vi "Get_Profile_paths.vi"(8 "error in (no error)":errorcluster, 10 "Target?":bool, 11 "OSArch":string) -> (0 "error out":errorcluster, 3 "profileDestPath":string)   [LabVIEW 2020, in "SEECD System Explorer.lvlib"]
uses:
  SEECD System Explorer.lvlib
  Applications/Utilities/ECAT Files.ctl
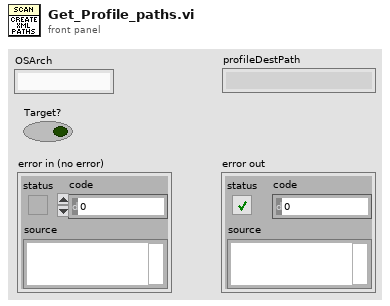
[diagram p1: front panel]
types:
  T1 = typedef "SEECD System Explorer.lvlib/ECAT Files.ctl" = enum16{"niECATLVProvider.mxx", "indcomecat.chm", "Providers DD", "Shared DD"}
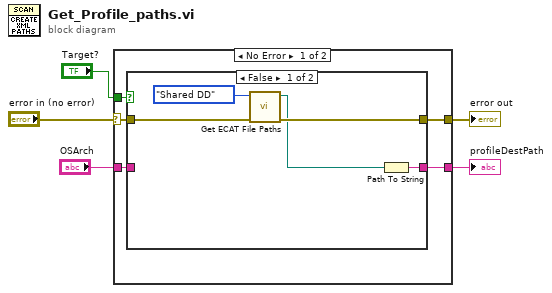
[diagram p0: block diagram]
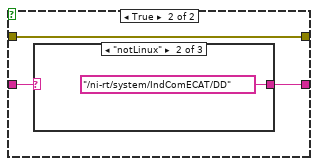
[diagram p2: hidden frame]
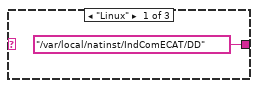
[diagram p3: hidden frame]
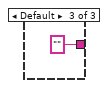
[diagram p4: hidden frame]
diagram:
  n1 = case shown="No Error" "error in (no error)" {
    selector: "error in (no error)" -> [w7 w22]
    tunnel: "OSArch" -> [w10 _]
    tunnel: [w6 w22] -> w4
    tunnel: "Target?" -> [w9 _]
    tunnel: [w8 _] -> w1
    frame No Error {
      n2 = case shown="False" w9 {
        tunnel: w10 -> [_ w18]
        tunnel: [w15 w17] -> w8
        tunnel: w7 -> [w14 w16]
        tunnel: [w13 w16] -> w6
        frame False {
          n3 = call "Get ECAT File Paths.vi"("error in"=w14, "ECAT File"=ECAT_Files."Shared DD") -> ("error out"=w13:errorcluster, "File Path"=w11:path)  [unwired: 8 in]
          n4 = Path To String(path=w11) -> (string=w15:string)
        }
        frame True {
          n5 = case shown="\"notLinux\"" w18 {
            tunnel: ["/var/local/natinst/IndComECAT/DD" "/ni-rt/system/IndComECAT/DD" ""] -> w17
            frame "Linux" {
            }
            frame "notLinux" {
            }
            frame Default {
            }
          }
        }
      }
    }
    frame Error {
    }
  }
  "error out" <- w4
  "profileDestPath" <- w1
